vi "pickup.vi"(10 "side":enum16{"l", "r"}(ring)) -> ()   [LabVIEW 2017]
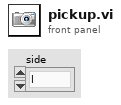
[diagram p1: front panel]
types:
  T1 = enum16{"hold", "f", "fl", "fr", "l", "r", "b", "bl", "br"}
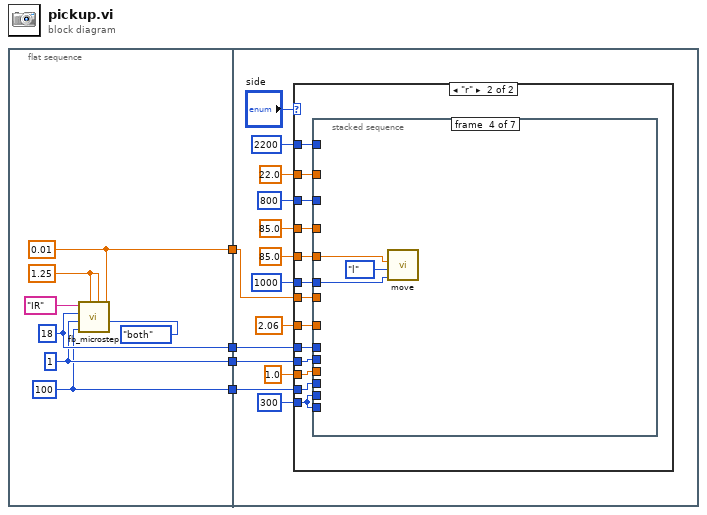
[diagram p0: block diagram]
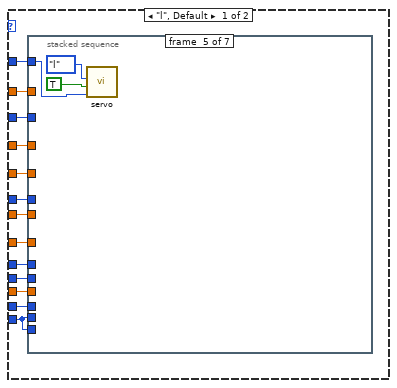
[diagram p2: hidden frame]
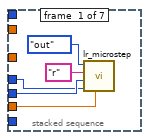
[diagram p3: hidden frame]
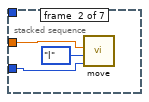
[diagram p4: hidden frame]
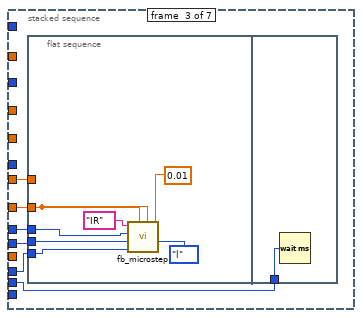
[diagram p5: hidden frame]
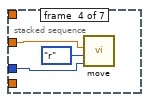
[diagram p6: hidden frame]
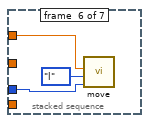
[diagram p7: hidden frame]
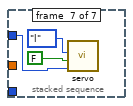
[diagram p8: hidden frame]
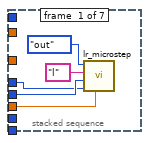
[diagram p9: hidden frame]
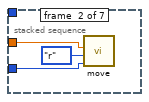
[diagram p10: hidden frame]
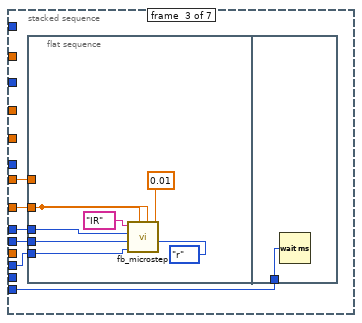
[diagram p11: hidden frame]
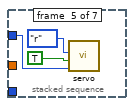
[diagram p12: hidden frame]
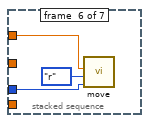
[diagram p13: hidden frame]
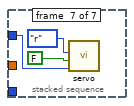
[diagram p14: hidden frame]
diagram:
  n1 = flat-sequence {
    tunnel: [w8] -> w4
    tunnel: [w7] -> w3
    tunnel: [w6] -> w2
    tunnel: [w5] -> w1
    tunnel: w4 -> [w25]
    tunnel: w3 -> [w24]
    tunnel: w2 -> [w23]
    tunnel: w1 -> [w22]
    frame #0 {
      w8 = 18 ("Delay")
      w7 = 1 ("Step")
      w6 = 100 ("SamplingNUM")
      w5 = 0.01 ("precision")
      w11 = 1.25 ("taget_IR_R")
      n2 = call "fb_microstep.vi"("Sensor"=enum16{"l", "r", "both"}."both", "precision"=w5, "taget_IR_L"=w11, "taget_IR_R"=w11, "SamplingNUM"=w6, "Step"=w7, "Delay"=w8, "Stop Mode"="IR") -> ()  [unwired: 3 in, 1 out]
    }
    frame #1 {
      n3 = case shown="\"r\"" "side" {
        tunnel: w25 -> [w38 w84]
        tunnel: w24 -> [w37 w83]
        tunnel: w23 -> [w36 w82]
        tunnel: w22 -> [w35 w85]
        tunnel: u32 2200 ("delay") -> [w30 w81]
        tunnel: u32 1000 ("milliseconds to wait") -> [w32 w80]
        tunnel: 85.0 ("D") -> [w31 w79]
        tunnel: 2.06 ("taget_IR_L") -> [w33 w78]
        tunnel: 1.0 ("logic_num") -> [w34 w77]
        tunnel: 85.0 ("D") -> [w29 w76]
        tunnel: 22.0 ("D") -> [w28 w75]
        tunnel: u32 800 ("milliseconds to wait") -> [w27 w74]
        tunnel: u32 300 ("milliseconds to wait") -> [w26 w73]
        frame "l", Default {
          n4 = stacked-sequence {
            tunnel: w38 -> [w39 _ w47 _ _ _ _]
            tunnel: w37 -> [w42 _ w52 _ _ _ _]
            tunnel: w36 -> [_ _ w51 _ _ _ _]
            tunnel: w35 -> [_ _ w50 _ _ _ _]
            tunnel: w34 -> [w41 _ _ _ _ _ _]
            tunnel: w33 -> [_ _ w49 _ _ _ _]
            tunnel: w32 -> [_ _ _ w61 _ w67 _]
            tunnel: w31 -> [_ _ _ w62 _ _ _]
            tunnel: w30 -> [_ _ _ _ w64 _ w70]
            tunnel: w29 -> [_ _ _ _ _ w68 _]
            tunnel: w28 -> [_ w46 _ _ _ _ _]
            tunnel: w27 -> [_ w44 _ _ _ _ _]
            tunnel: w26 -> [_ _ _ _ _ _ _]
            tunnel: w26 -> [_ _ w48 _ _ _ _]
            frame #0 {
              n5 = call "lr_microstep.vi"("target_IR"=w41, "Delay"=w39, "Step"=w42, "Stop Mode"="r", "IN-OUT"=enum16{"out", "in"}."out") -> ()  [unwired: 6 in, 1 out]
            }
            frame #1 {
              n6 = call "move.vi"("delay"=w44, "Enum"=T1."l", "D"=w46) -> ()  [unwired: 9 in]
            }
            frame #2 {
              n7 = flat-sequence {
                tunnel: w52 -> [w57]
                tunnel: w51 -> [w56]
                tunnel: w50 -> [_]
                tunnel: w49 -> [w54]
                tunnel: w47 -> [w53]
                tunnel: w48 -> [w60]
                frame #0 {
                  n8 = call "fb_microstep.vi"("Sensor"=enum16{"l", "r", "both"}."l", "precision"=0.01, "taget_IR_L"=w54, "taget_IR_R"=w54, "SamplingNUM"=w56, "Step"=w57, "Delay"=w53, "Stop Mode"="IR") -> ()  [unwired: 3 in, 1 out]
                }
                frame #1 {
                  n9 = Wait (ms)(milliseconds to wait=w60) -> ()  [unwired: 1 out]
                }
              }
            }
            frame #3 {
              n10 = call "move.vi"("delay"=w61, "Enum"=T1."r", "D"=w62) -> ()  [unwired: 9 in]
            }
            frame #4 {
              n11 = call "servo.vi"("delay"=w64, "in=true\nout = false"=TRUE ("in=true\nout = false"), "left-right"=enum16{"r", "l"}."l") -> ()  [unwired: 9 in]
            }
            frame #5 {
              n12 = call "move.vi"("delay"=w67, "Enum"=T1."l", "D"=w68) -> ()  [unwired: 9 in]
            }
            frame #6 {
              n13 = call "servo.vi"("delay"=w70, "in=true\nout = false"=FALSE ("in=true\nout = false"), "left-right"=enum16{"r", "l"}."l") -> ()  [unwired: 9 in]
            }
          }
        }
        frame "r" {
          n14 = stacked-sequence {
            tunnel: w85 -> [_ _ w99 _ _ _ _]
            tunnel: w84 -> [w86 _ w94 _ _ _ _]
            tunnel: w83 -> [w89 _ w98 _ _ _ _]
            tunnel: w82 -> [_ _ w97 _ _ _ _]
            tunnel: w77 -> [w88 _ _ _ _ _ _]
            tunnel: w78 -> [_ _ w96 _ _ _ _]
            tunnel: w80 -> [_ _ _ w108 _ w114 _]
            tunnel: w79 -> [_ _ _ w109 _ _ _]
            tunnel: w81 -> [_ _ _ _ w111 _ w117]
            tunnel: w76 -> [_ _ _ _ _ w115 _]
            tunnel: w75 -> [_ w92 _ _ _ _ _]
            tunnel: w74 -> [_ w91 _ _ _ _ _]
            tunnel: w73 -> [_ _ _ _ _ _ _]
            tunnel: w73 -> [_ _ w95 _ _ _ _]
            frame #0 {
              n15 = call "lr_microstep.vi"("target_IR"=w88, "Delay"=w86, "Step"=w89, "Stop Mode"="l", "IN-OUT"=enum16{"out", "in"}."out") -> ()  [unwired: 6 in, 1 out]
            }
            frame #1 {
              n16 = call "move.vi"("delay"=w91, "Enum"=T1."r", "D"=w92) -> ()  [unwired: 9 in]
            }
            frame #2 {
              n17 = flat-sequence {
                tunnel: w99 -> [_]
                tunnel: w98 -> [w104]
                tunnel: w97 -> [w103]
                tunnel: w96 -> [w102]
                tunnel: w94 -> [w101]
                tunnel: w95 -> [w107]
                frame #0 {
                  n18 = call "fb_microstep.vi"("Sensor"=enum16{"l", "r", "both"}."r", "precision"=0.01, "taget_IR_L"=w102, "taget_IR_R"=w102, "SamplingNUM"=w103, "Step"=w104, "Delay"=w101, "Stop Mode"="IR") -> ()  [unwired: 3 in, 1 out]
                }
                frame #1 {
                  n19 = Wait (ms)(milliseconds to wait=w107) -> ()  [unwired: 1 out]
                }
              }
            }
            frame #3 {
              n20 = call "move.vi"("delay"=w108, "Enum"=T1."l", "D"=w109) -> ()  [unwired: 9 in]
            }
            frame #4 {
              n21 = call "servo.vi"("delay"=w111, "in=true\nout = false"=TRUE ("in=true\nout = false"), "left-right"=enum16{"r", "l"}."r") -> ()  [unwired: 9 in]
            }
            frame #5 {
              n22 = call "move.vi"("delay"=w114, "Enum"=T1."r", "D"=w115) -> ()  [unwired: 9 in]
            }
            frame #6 {
              n23 = call "servo.vi"("delay"=w117, "in=true\nout = false"=FALSE ("in=true\nout = false"), "left-right"=enum16{"r", "l"}."r") -> ()  [unwired: 9 in]
            }
          }
        }
      }
    }
  }
